vi "ClosePage.vi"(7 "popup viewer":bool, 8 "Fehler (Eingang, kein Fehler)":errorcluster, 11 "Context (Eingang)":refnum<class "Context.lvclass">) -> (0 "Fehler (Ausgang)":errorcluster)   [LabVIEW 2020, in "PDF Interface.lvlib"]
doc: "Close the PDF created by \"InitBeforePage\" and after added content and optional addtional pages finished."
uses:
  PDF Interface.lvlib
  <vilib>/Simplicity AI/SAI_PDF_API/Classes/Context/Context.lvclass
  <vilib>/Simplicity AI/SAI_PDF_API/SAI_PDF_Toolkit.lvlib
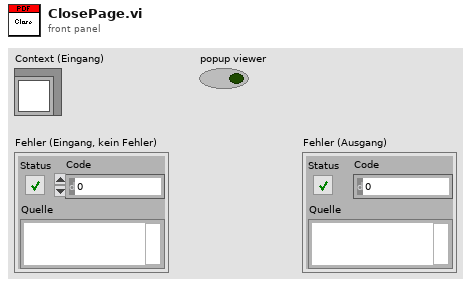
[diagram p1: front panel]
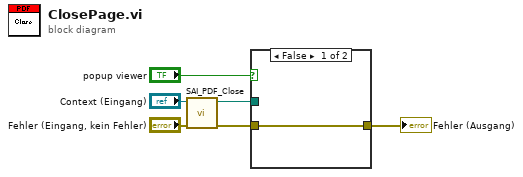
[diagram p0: block diagram]
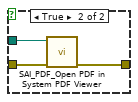
[diagram p2: hidden frame]
diagram:
  n1 = call <vilib>:"SAI_PDF_Close.vi"("error in"="Fehler (Eingang, kein Fehler)", "Context In"="Context (Eingang)") -> ("error out"=w2:errorcluster, "Path"=w3:path)  [unwired: 8 out]
  n2 = case shown="False" "popup viewer" {
    tunnel: [w7 w10] -> w4
    tunnel: w3 -> [_ w9]
    tunnel: w2 -> [w7 w8]
    frame False {
    }
    frame True {
      n3 = call <vilib>:"SAI_PDF_Open PDF in System PDF Viewer.vi"("error in"=w8, "Path"=w9) -> ("error out"=w10:errorcluster)  [unwired: 9 out]
    }
  }
  "Fehler (Ausgang)" <- w4
